vi "Read Container.vi"(8 "error in (no error)":errorcluster, 10 "Sample Line (All Closed)":T2, 11 "Sample Line in":refnum<class "Sample Line.lvclass">) -> (0 "error out":errorcluster, 1 "Sample":refnum<class "Sample.lvclass">, 2 "Containers":T1[](array[typedef]), 3 "Sample Line out":refnum<class "Sample Line.lvclass">)   [LabVIEW 2015, in "cRIO-Carbondioxide.lvlib" / "CO2-Actor.lvlib" / "Sample Line.lvclass"]
uses:
  Sample Line.lvclass
  Controls/Sample Line State Enumerator.ctl
  subs/Sample/Sample.lvclass
  Controls/Sample Container.ctl
  Sample Line.lvclass/Sample Line.ctl
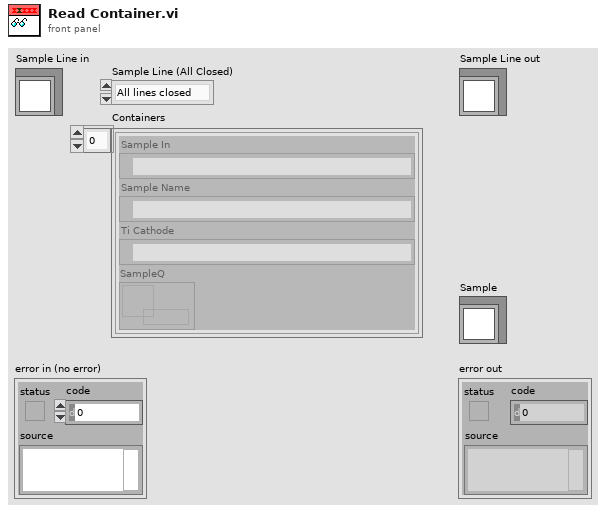
[diagram p1: front panel]
types:
  T1 = typedef "Sample Container.ctl" = cluster{"Sample In":refnum<k21>, "Sample Name":refnum<k21>, "Ti Cathode":refnum<k21>, "SampleQ":refnum<queue>}
  T2 = typedef "Sample Line State Enumerator.ctl" = enum16{"All lines closed", "Sample line 1.", "Sample line 2.", "Sample line 3.", "Sample line 4.", "Sample line 5.", "Out of range"}
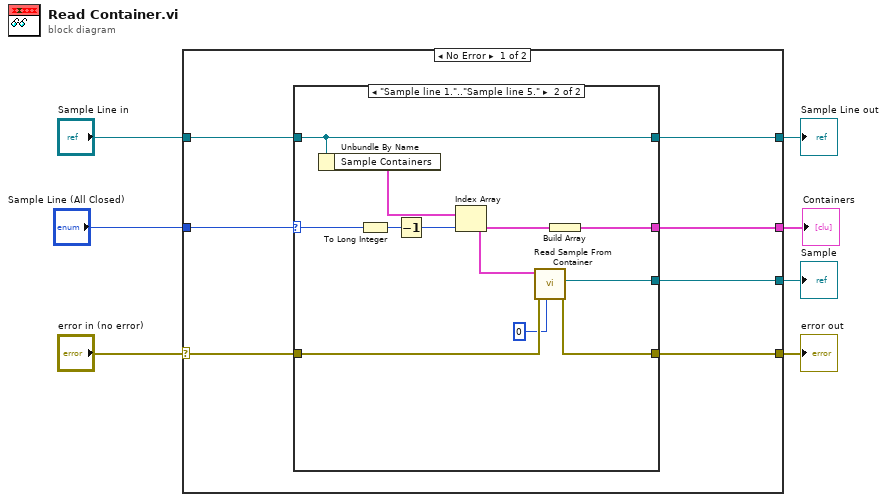
[diagram p0: block diagram]
diagram:
  n1 = case shown="No Error" "error in (no error)" {
    selector: "error in (no error)" -> [w12 w29]
    tunnel: [w11 w29] -> w6
    tunnel: [w10 w28] -> w4
    tunnel: "Sample Line in" -> [w13 w28]
    tunnel: "Sample Line (All Closed)" -> [w14 _]
    tunnel: [w9 _] -> w2
    tunnel: [w8 _] -> w1
    frame No Error {
      n2 = case shown="\"Sample line 1.\"..\"Sample line 5.\"" w14 {
        selector: w14 -> [_ w26]
        tunnel: w13 -> [w16 w27]
        tunnel: w12 -> [w15 w22]
        tunnel: [w15 w21] -> w11
        tunnel: [w16 w27] -> w10
        tunnel: [_ w17] -> w8
        tunnel: [_ w20] -> w9
        frame "All lines closed", Default {
        }
        frame "Sample line 1.".."Sample line 5." {
          n3 = Unbundle By Name(w27) -> ("Sample Containers"=w23:T1[])
          n4 = To Long Integer(number=w26) -> (32bit integer=w25:i32)
          n5 = Decrement(x=w25) -> (x-1=w24:i32)
          n6 = Index Array(array=w23, index=w24) -> (element=w19:T1)
          n7 = call "Read Sample From Container.vi"("Queue timeout in ms (-1)"=0 ("timeout in ms (-1)"), "error in (no error)"=w22, "Container"=w19) -> ("error out"=w21:errorcluster, "Sample out"=w20:refnum<class "Sample.lvclass">)  [unwired: 4 in, 3 out]
          n8 = Build Array(w19) -> (w17:T1[])
        }
      }
    }
    frame Error {
    }
  }
  "error out" <- w6
  "Sample Line out" <- w4
  "Sample" <- w2
  "Containers" <- w1
